vi "PRIME Detector Object Test Program.vi"(8 "error in (no error)":errorcluster) -> (0 "error out":errorcluster)   [LabVIEW 2020]
uses:
  RIMAS Detector Config.ctl
  RIMAS Detector Server Config.ctl
  RIMAS Observation Config.ctl
  Detector enum Detector Integration Mode.ctl
  PRIME Detector.lvclass
  PRIME Detector.lvclass/PRIME Detector.ctl
panel:
  in  "Init?":bool
  in  "Exposure Time":dbl
  in  "Detector Config":T1={"Detector"=0, "Offsets"=[[0, 0, 0, 0, 0, 0, 0, 0, 0, 0, 0, 0, 0, 0, 0, 0, 0, 0, 0, 0, 0, 0, 0, 0, 0, 0, 0, 0, 0, 0, 0, 0]], "Detector Computer"={"Machine"="192.168.121.11", "Password"="", "FITS File Path"="", "Port"=44444, "Header Path"="", "Name"=""}, "FITS hdr template0"=path "", "FITS hdr template1"=path "", "FITS Data File Path"=path "", "FITS Detector Settings"={"Exp Time Short"=0.0, "# of Frames"=0.0, "Exp Time Long"=0.0, "# of Groups"=0.0, "Object Name"="", "Object"="", "Obs Type"="", "Image Type"="", "Observer"="", "Observer Affiliation"=""}, "Sim Folder"=path "", "Integration Mode"=enum."SSR", "Integration Time"=0.0, "Frame Int Time"=0.0} {"Offsets" format="%04x"; "Detector" items=["0", "1", "2"]}
  # "sec"
  # "sec"
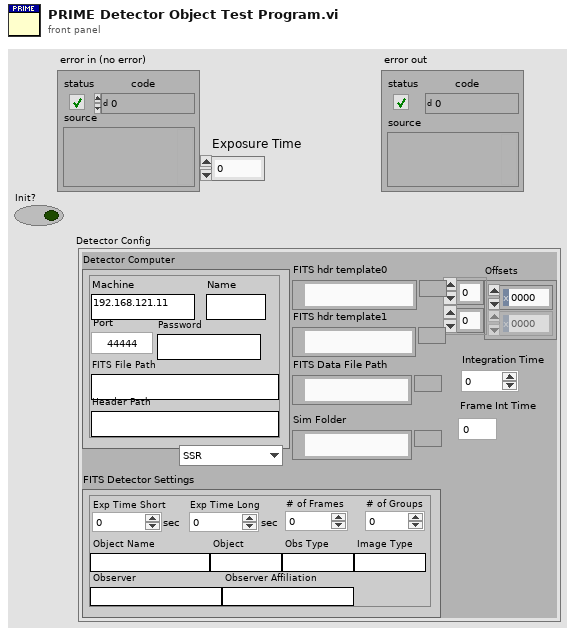
[diagram p1: front panel]
types:
  T1 = typedef "RIMAS Detector Config.ctl" = cluster{"Detector":u16, "Offsets":u16[][], "Detector Computer":T2, "FITS hdr template0":path, "FITS hdr template1":path, "FITS Data File Path":path, "FITS Detector Settings":T3, "Sim Folder":path, "Integration Mode":T4, "Integration Time":dbl, "Frame Int Time":dbl}
  T2 = typedef "RIMAS Detector Server Config.ctl" = cluster{"Machine":string, "Password":string, "FITS File Path":string, "Port":u16, "Header Path":string, "Name":string}
  T3 = typedef "RIMAS Observation Config.ctl" = cluster{"Exp Time Short":dbl, "# of Frames":dbl, "Exp Time Long":dbl, "# of Groups":dbl, "Object Name":string, "Object":string, "Obs Type":string, "Image Type":string, "Observer":string, "Observer Affiliation":string}
  T4 = typedef "Detector enum Detector Integration Mode.ctl" = enum16{"SSR", "CDS", "MEAN", "MEDIAN", "MODE", "MIIN", "MAX"}
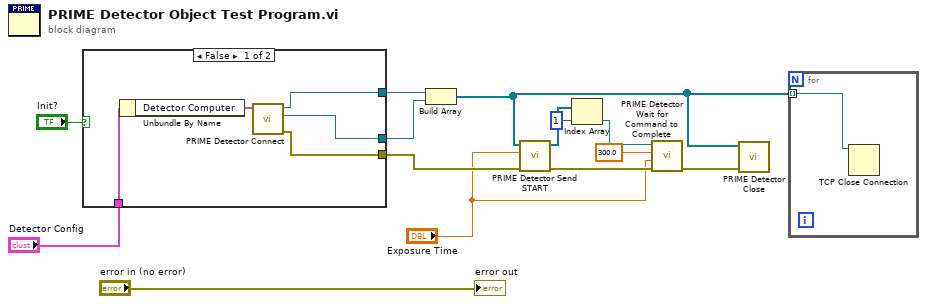
[diagram p0: block diagram]
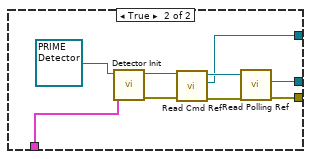
[diagram p2: hidden frame]
diagram:
  n1 = case shown="False" "Init?" {
    tunnel: "Detector Config" -> [w16 w27]
    tunnel: [w19 w24] -> w10
    tunnel: [w18 w23] -> w9
    tunnel: [w17 w20] -> w8
    frame False {
      n2 = Unbundle By Name(w16) -> ("Detector Computer"=w15:T2)
      n3 = call "PRIME Detector Connect.vi"("Detector Computer"=w15) -> ("error out"=w17:errorcluster, "Polling Ref"=w18:refnum<k5>, "Cmd Ref"=w19:refnum<k5>)  [unwired: 7 in, 1 out]
    }
    frame True {
      n4 = call-dynamic "Detector Init.vi"("Detector Config"=w27, "PRIME Detector in"=refnum<class "PRIME Detector.lvclass"> refnum ("PRIME Detector.lvclass")) -> ("error out"=w22:errorcluster, "PRIME Detector out"=w26:refnum<class "PRIME Detector.lvclass">)  [unwired: 7 in, 1 out]
      n5 = call "Read Cmd Ref.vi"("error in (no error)"=w22, "PRIME Detector in"=w26) -> ("error out"=w21:errorcluster, "Cmd Ref"=w24:refnum<k5>, "PRIME Detector out"=w25:refnum<class "PRIME Detector.lvclass">)  [unwired: 7 in]
      n6 = call "Read Polling Ref.vi"("error in (no error)"=w21, "PRIME Detector in"=w25) -> ("error out"=w20:errorcluster, "Polling Ref"=w23:refnum<k5>)  [unwired: 7 in, 1 out]
    }
  }
  n7 = Build Array(w10, w9) -> (w3:refnum<k5>[])
  n8 = call "PRIME Detector Send START.vi"("error in (no error)"=w8, "Exposure Time"="Exposure Time", "connection ID"=w3) -> ("error out"=w12:errorcluster, "connection ID out"=w7:refnum<k5>[])  [unwired: 7 in]
  n9 = Index Array(array=w7, index=1) -> (element=w5:refnum<k5>)
  n10 = call "PRIME Detector Wait for Command to Complete.vi"("error in (no error)"=w12, "Exp Time"="Exposure Time", "timeout (120s)"=300.0, "connection ID"=w5) -> ("error out"=w4:errorcluster)  [unwired: 5 in, 2 out]
  n11 = call "PRIME Detector Close.vi"("error in (no error)"=w4, "connection ID"=w3) -> ()  [unwired: 8 in, 2 out]
  n12 = for {
    tunnel: w3 -> [w29] mode=indexing
    n13 = TCP Close Connection(connection ID=w29) -> ()  [unwired: 2 in, 2 out]
  }
  "error out" <- "error in (no error)"
